vi "CS++DMM-Synchronized-Readout.vi"() -> ()   [LabVIEW 2016, in "CS++DMM.lvlib"]
uses:
  CS++DMM.lvlib
  CSPP_Core/Classes/CS++BaseClasses/Factory/CS++Factory.lvclass
  CSPP_Core/Classes/CS++BaseClasses/Factory/CS++Factory.lvclass/CS++Factory.ctl
  CS++DMM.lvclass
  C:/User/Brand/LVP/CSPP-Dev/Packages/CSPP_Core/Actors/CS++DeviceActor/CS++DeviceActor.lvclass
  CSPP_Core/Actors/CS++DeviceActor/CS++DeviceActor.lvclass/CS++DeviceActor.ctl
  CSPP_Core/Actors/CS++DeviceActor/Read Resource Name.vi
  CSPP_Core/Actors/CS++DeviceActor/CS++DeviceActor.lvclass
panel:
  in  "Trigger Delays":dbl[unit][](array[numeric])=[0.0, 0.0] format="%.3f"
  out "dt":dbl[unit] format="%.3f"
  out "Apertures":dbl[unit][](array[numeric])
  out "Samples":i32[](array[numeric])
  out "Graph":cluster{dbl[unit][]}[](graph)
  in  "Sample count":i32=10 caption="sample count (1)"
  in  "Sample Frequency":dbl[unit]=1.0 caption="sample interval (0.0 s)" format="%.3f"
  in  "CS++Object Names":string[](array[string])=["DMM3458A-GPIB0-21", "DMM3458A-GPIB0-22"]
  in  "File Path Control":path=path "C:/User/Brand/LVP/STF/STF.ini"
  out "error out":errorcluster
  in  "Stop":bool
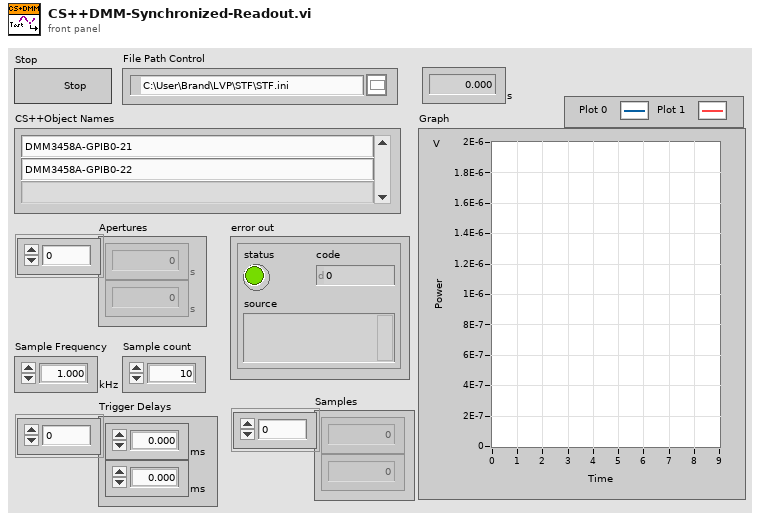
[diagram p1: front panel]
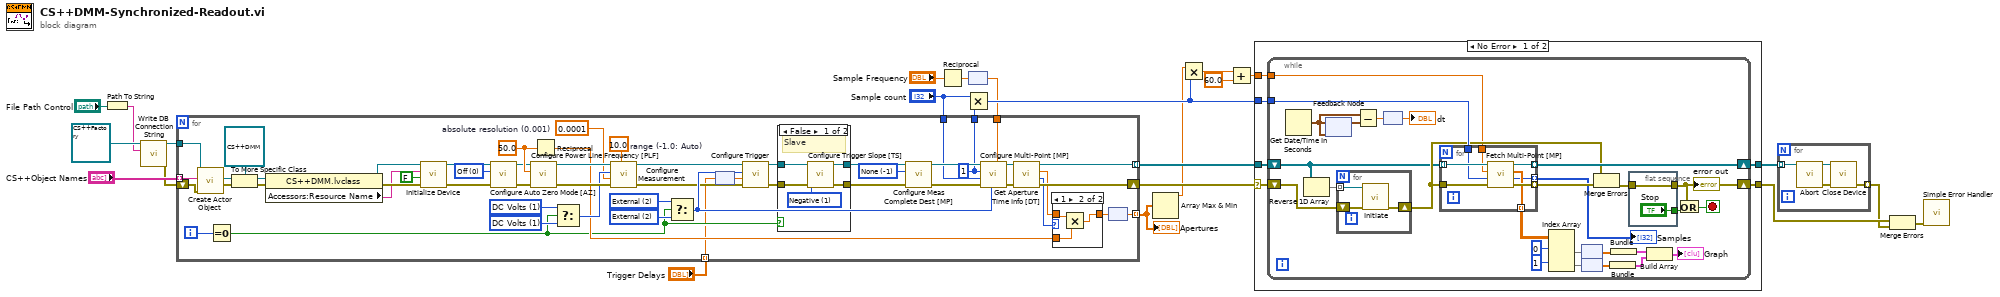
[diagram p0: block diagram]
diagram:
  n1 = Path To String(path="File Path Control") -> (string=w19:string)
  n2 = call "Write DB Connection String.vi"("DB Connection String"=w19, "CS++Factory in"=refnum<class "CS++Factory.lvclass"> refnum ("CS++BaseClasses.lvlib:CS++Factory.lvclass")) -> ("error out"=w14:errorcluster, "CS++Factory out"=w21:refnum<class "CS++Factory.lvclass">)  [unwired: 8 in]
  n3 = Reciprocal(x="Sample Frequency") -> (1/x=w3:dbl[unit])
  n4 = node(w3) -> (w7:dbl)
  n5 = for {
    tunnel: w21 -> [w77]
    tunnel: "CS++Object Names" -> [w72] mode=indexing
    tunnel: [w57] -> w24 mode=indexing
    shift-right: [w56] -> w5
    shift-left: w14 -> [w66]
    tunnel: "Sample count" -> [w27]
    tunnel: w7 -> [w55]
    tunnel: [w49] -> w4 mode=indexing
    tunnel: [w36] -> w10
    tunnel: "Trigger Delays" -> [w35] mode=indexing
    i -> [w33]
    w28 = 0.0001  # absolute resolution (0.001)
    w29 = 0 items=["On"=1, "Off"=0, "Once"=2] ("auto zero mode (Off)")
    w32 = 10.0  # range (-1.0: Auto)
    w58 = -1 items=["None"=-1, "External"=2, "PXI TRIG0 or VXI TTL0"=111, "PXI TRIG1 or VXI TTL1"=112, "PXI TRIG2 or VXI TTL2"=113, "PXI TRIG3 or VXI TTL3"=114, "PXI TRIG4 or VXI TTL4"=115, "PXI TRIG5 or VXI TTL5"=116, "PXI TRIG6 or VXI TTL6"=117, "PXI TRIG7 or VXI TTL7"=118, "ECL0"=119, "ECL1"=120, "PXI Star"=131, "RTSI 0"=140, "RTSI 1"=141, "RTSI 2"=142, "RTSI 3"=143, "RTSI 4"=144, "RTSI 5"=145, "RTSI 6"=146] ("meas complete dest (None)")
    w59 = 2 items=["Immediate"=1, "External"=2, "Software Trigger Function"=3, "Interval"=10, "PXI TRIG0 or VXI TTL0"=111, "PXI TRIG1 or VXI TTL1"=112, "PXI TRIG2 or VXI TTL2"=113, "PXI TRIG3 or VXI TTL3"=114, "PXI TRIG4 or VXI TTL4"=115, "PXI TRIG5 or VXI TTL5"=116, "PXI TRIG6 or VXI TTL6"=117, "PXI TRIG7 or VXI TTL7"=118, "ECL0"=119, "ECL1"=120, "PXI Star"=131, "RTSI 0"=140, "RTSI 1"=141, "RTSI 2"=142, "RTSI 3"=143, "RTSI 4"=144, "RTSI 5"=145, "RTSI 6"=146] ("sample trigger (Immediate)")
    w60 = 2 items=["Immediate"=1, "External"=2, "Software Trigger Function"=3, "Interval"=10, "PXI TRIG0 or VXI TTL0"=111, "PXI TRIG1 or VXI TTL1"=112, "PXI TRIG2 or VXI TTL2"=113, "PXI TRIG3 or VXI TTL3"=114, "PXI TRIG4 or VXI TTL4"=115, "PXI TRIG5 or VXI TTL5"=116, "PXI TRIG6 or VXI TTL6"=117, "PXI TRIG7 or VXI TTL7"=118, "ECL0"=119, "ECL1"=120, "PXI Star"=131, "RTSI 0"=140, "RTSI 1"=141, "RTSI 2"=142, "RTSI 3"=143, "RTSI 4"=144, "RTSI 5"=145, "RTSI 6"=146] ("sample trigger (Immediate)")
    w36 = 1 ("trigger count (1)")
    w61 = 1 items=["DC Volts"=1, "AC Volts"=2, "DC Current"=3, "AC Current"=4, "2 Wire Resistance"=5, "4 Wire Resistance"=101, "AC + DC Volts"=106, "AC + DC Current"=107, "Frequency"=104, "Period"=105, "Temperature"=108] ("measurement function (DC Volts)")
    w63 = 1 items=["DC Volts"=1, "AC Volts"=2, "DC Current"=3, "AC Current"=4, "2 Wire Resistance"=5, "4 Wire Resistance"=101, "AC + DC Volts"=106, "AC + DC Current"=107, "Frequency"=104, "Period"=105, "Temperature"=108] ("measurement function (DC Volts)")
    w51 = 50.0 ("power line frequency (60.0 Hz)")
    n6 = call "Create Actor Object.vi"("error in (no error)"=w66, "Object Name"=w72, "CS++Factory in"=w77) -> ("error out"=w75:errorcluster, "CS++BaseActor"=w76:refnum<class "CS++BaseActor.lvclass">)  [unwired: 5 in, 2 out]
    n7 = Equal To 0?(x=w33) -> (x = 0?=w46:bool)
    n8 = To More Specific Class(target class=refnum<class "CS++DMM.lvclass"> refnum ("CS++DMM.lvlib:CS++DMM.lvclass"), reference=w76, error in=w75) -> (specific class reference=w73:refnum<class "CS++DMM.lvclass">, error out=w70:errorcluster)
    n9 = property class="CS++DMM.lvclass"(reference=w73, error in=w70) -> (reference out=w71:refnum<class "CS++DMM.lvclass">, error out=w69:errorcluster, "Accessors:Resource Name"=w68:string)
    n10 = call "Initialize Device.vi"("error in (no error)"=w69, "Reset (F)"=FALSE, "Resource Name"=w68, "CS++DeviceActor in"=w71) -> ("error out"=w25:errorcluster, "CS++DeviceActor out"=w26:refnum<class "CS++DMM.lvclass">)  [unwired: 6 in]
    n11 = call "Configure Auto Zero Mode [AZ].vi"("error in (no error)"=w25, "auto zero mode (Off)"=w29, "CS++DMM in"=w26) -> ("error out"=w30:errorcluster, "CS++DMM out"=w31:refnum<class "CS++DMM.lvclass">)  [unwired: 7 in]
    n12 = call "Configure Power Line Frequency [PLF].vi"("error in (no error)"=w30, "power line frequency (60.0 Hz)"=w51, "CS++DMM in"=w31) -> ("error out"=w64:errorcluster, "CS++DMM out"=w65:refnum<class "CS++DMM.lvclass">)  [unwired: 7 in]
    n13 = Reciprocal(x=w51) -> (1/x=w50:dbl)
    n14 = Select(t=w63, s=w46, f=w61) -> (s? t:f=w62:i32)
    n15 = call "Configure Measurement.vi"("range (-1.0: Auto)"=w32, "error in (no error)"=w64, "absolute resolution (0.001)"=w28, "measurement function (DC Volts)"=w62, "CS++DMM in"=w65) -> ("error out"=w41:errorcluster, "CS++DMM out"=w42:refnum<class "CS++DMM.lvclass">)  [unwired: 5 in]
    n16 = Select(t=w60, s=w46, f=w59) -> (s? t:f=w43:i32)
    n17 = node(w35) -> (w34:dbl)
    n18 = call "Configure Trigger.vi"("error in (no error)"=w41, "trigger delay (0.0 s)"=w34, "trigger source (Immediate)"=w43, "CS++DMM in"=w42) -> ("error out"=w44:errorcluster, "CS++DMM out"=w45:refnum<class "CS++DMM.lvclass">)  [unwired: 6 in]
    n19 = case shown="False" w46 {
      tunnel: w45 -> [w82 w84]
      tunnel: [w81 w84] -> w48
      tunnel: w44 -> [w80 w83]
      tunnel: [w79 w83] -> w47
      frame False {
        w78 = 1 items=["Positive", "Negative"] ("trigger slope (0: Positive)")
        # "Slave"
        n20 = call "Configure Trigger Slope [TS].vi"("error in (no error)"=w80, "trigger slope (0: Positive)"=w78, "CS++DMM in"=w82) -> ("error out"=w79:errorcluster, "CS++DMM out"=w81:refnum<class "CS++DMM.lvclass">)  [unwired: 7 in]
      }
      frame True {
        # "Master"
      }
    }
    n21 = call "Configure Meas Complete Dest [MP].vi"("error in (no error)"=w47, "meas complete dest (None)"=w58, "CS++DMM in"=w48) -> ("error out"=w39:errorcluster, "CS++DMM out"=w40:refnum<class "CS++DMM.lvclass">)  [unwired: 7 in]
    n22 = call "Configure Multi-Point [MP].vi"("sample interval (0.0 s)"=w55, "sample trigger (Immediate)"=w43, "error in (no error)"=w39, "sample count (1)"=w27, "trigger count (1)"=w36, "CS++DMM in"=w40) -> ("error out"=w37:errorcluster, "CS++DMM out"=w38:refnum<class "CS++DMM.lvclass">)  [unwired: 4 in]
    n23 = call "Get Aperture Time Info [DT].vi"("error in (no error)"=w37, "CS++DMM in"=w38) -> ("error out"=w56:errorcluster, "aperture time units"=w54:i32, "aperture time (sec)"=w53:dbl, "CS++DMM out"=w57:refnum<class "CS++DMM.lvclass">)  [unwired: 6 in]
    n24 = case shown="1" w54 {
      tunnel: w53 -> [w85 w88]
      tunnel: [w85 w86] -> w52
      tunnel: w50 -> [_ w87]
      frame 0, Default {
      }
      frame 1 {
        n25 = Multiply(x=w88, y=w87) -> (x*y=w86:dbl)
      }
    }
    n26 = node(w52) -> (w49:dbl[unit])
  }
  "Apertures" <- w4
  n27 = Multiply(x="Sample count", y=w10) -> (x*y=w9:i32)
  n28 = Array Max & Min(array=w4) -> (max value=w2:dbl[unit])  [unwired: 3 out]
  n29 = Multiply(x=w2, y=w9) -> (x*y=w13:dbl[unit])
  n30 = Add(x=w13, y=dbl[unit] 60.0 ("x")) -> (x+y=w11:dbl[unit])
  n31 = case shown="No Error" w5 {
    selector: w5 -> [w93 w135]
    tunnel: w24 -> [w94 w136]
    tunnel: [w92 w136] -> w23
    tunnel: [w91 w135] -> w18
    tunnel: w11 -> [w90 _]
    tunnel: w9 -> [w89 _]
    frame No Error {
      n32 = while {
        shift-right: [w103] -> w91
        shift-left: w93 -> [w121]
        shift-right: [w119] -> w92
        shift-left: w94 -> [w105]
        tunnel: w90 -> [w104]
        tunnel: w89 -> [w118]
        stop <- w113 stop-if-true
        n33 = Get Date/Time In Seconds() -> (seconds since 1Jan1904=w110:timestamp)
        n34 = Reverse 1D Array(array=w105) -> (reversed array=w101:refnum<class "CS++DMM.lvclass">[])
        n35 = feedback #1(w110) -> (w109:timestamp)
        n36 = feedback-in #1(w110) -> ()
        n37 = for {
          tunnel: w101 -> [w124] mode=indexing
          shift-right: [w122] -> w106
          shift-left: w121 -> [w123]
          n38 = call "Initiate.vi"("error in (no error)"=w123, "CS++DMM in"=w124) -> ("error out"=w122:errorcluster)  [unwired: 8 in, 1 out]
        }
        n39 = Subtract(x=w110, y=w109) -> (x-y=w108:dbl)
        n40 = node(w108) -> (→"dt":dbl[unit])
        n41 = for {
          tunnel: w105 -> [w134] mode=indexing
          tunnel: [w133] -> w119 mode=indexing
          tunnel: w118 -> [w127]
          tunnel: [w131] -> w100 mode=indexing
          tunnel: [w130] -> w111 mode=indexing
          tunnel: w104 -> [w129]
          tunnel: [w132] -> w112 mode=indexing
          tunnel: w106 -> [w128]
          n42 = call "Fetch Multi-Point [MP].vi"("error in (no error)"=w128, "array size"=w127, "maximum time (5s)"=w129, "CS++DMM in"=w134) -> ("error out"=w132:errorcluster, "actual number of points"=w130:i32, "reading array"=w131:dbl[], "CS++DMM out"=w133:refnum<class "CS++DMM.lvclass">)  [unwired: 4 in]
        }
        "Samples" <- w111
        n43 = Index Array(array=w100, index (row) #1=0 ("index (row)"), index (row) #2=1 ("index (row)")) -> (element #1=w115:dbl[], element #2=w114:dbl[])  [unwired: 2 in]
        n44 = node(w115) -> (w99:dbl[unit][])
        n45 = node(w114) -> (w98:dbl[unit][])
        n46 = Merge Errors(w106, w112) -> (w102:errorcluster)
        n47 = Bundle(w98) -> (w96:cluster{dbl[unit][]})  [unwired: 1 in]
        n48 = Bundle(w99) -> (w97:cluster{dbl[unit][]})  [unwired: 1 in]
        n49 = flat-sequence {
          tunnel: ["Stop"] -> w120
          tunnel: [w125] -> w103
          tunnel: w102 -> [w125]
          frame #0 {
          }
        }
        n50 = Build Array(w97, w96) -> (→"Graph":cluster{dbl[unit][]}[])
        n51 = Or(x=w103, y=w120) -> (x .or. y?=w113:bool)
        "error out" <- w103
      }
    }
    frame Error {
    }
  }
  n52 = for {
    tunnel: w23 -> [w139] mode=indexing
    tunnel: [w140] -> w17 mode=indexing
    n53 = call "Abort.vi"("CS++DMM in"=w139) -> ("error out"=w137:errorcluster, "CS++DMM out"=w138:refnum<class "CS++DMM.lvclass">)  [unwired: 9 in]
    n54 = call "Close Device.vi"("error in (no error)"=w137, "CS++DeviceActor in"=w138) -> ("error out"=w140:errorcluster)  [unwired: 8 in, 1 out]
  }
  n55 = Merge Errors(w18, w17) -> (w16:errorcluster)
  n56 = call <vilib>:"Simple Error Handler.vi"("error in (no error)"=w16) -> ()  [unwired: 4 in, 5 out]
